vi "Write Device Name.vi"(8 "error in (no error)":errorcluster, 10 "device name":string, 11 "PLBB in":refnum<class "PL BlackBox Modbus Client.lvclass">) -> (0 "error out":errorcluster, 3 "PLBB out":refnum<class "PL BlackBox Modbus Client.lvclass">)   [LabVIEW 2015, in "PL BlackBox Modbus Client.lvclass"]
doc: "Writes the device name."
uses:
  PL BlackBox Modbus Client.lvclass
  <vilib>/plasmapper/PL Modbus Client/PL Modbus Client.lvclass
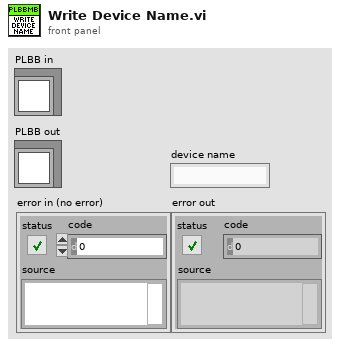
[diagram p1: front panel]
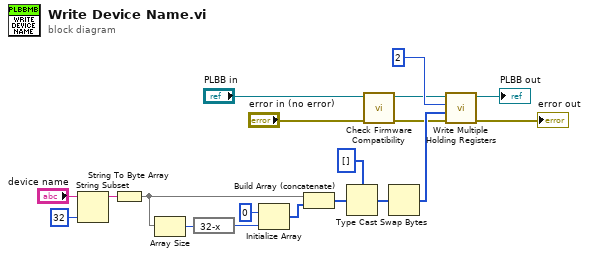
[diagram p0: block diagram]
diagram:
  n1 = String Subset(string="device name", length (rest)=32 ("length (rest)")) -> (substring=w10:string)  [unwired: 1 in]
  n2 = String To Byte Array(string=w10) -> (unsigned byte array=w14:u8[])
  n3 = Array Size(array=w14) -> (size(s)=w8:i32)
  n4 = expression code="32-x"(w8) -> (w7:i32)
  n5 = Initialize Array(u8 0, w7) -> (w15:u8[])
  n6 = Build Array (concatenate)(w14, w15) -> (w11:u8[])
  n7 = Type Cast(type=u16[] [] ("values"), x=w11) -> (*(type *) &x=w12:u16[])
  n8 = call-dynamic "Check Firmware Compatibility.vi"("error in (no error)"="error in (no error)", "PLBB in"="PLBB in") -> ("error out"=w3:errorcluster, "PLBB out"=w4:refnum<class "PL BlackBox Modbus Client.lvclass">)  [unwired: 8 in]
  n9 = Swap Bytes(anything=w12) -> (byte swapped=w5:u16[])
  n10 = call <vilib>:"Write Multiple Holding Registers.vi"("error in (no error)"=w3, "values"=w5, "address"=u16 2, "MODBUS in"=w4) -> ("error out"=→"error out":errorcluster, "MODBUS out"=→"PLBB out":refnum<class "PL BlackBox Modbus Client.lvclass">)  [unwired: 6 in]
